vi "Lockstep Move.vi"(6 "Movement Type (0: relative)":u16(ring) items=["relative", "absolute"], 7 "Move Distance (0)":i32, 8 "error in (no error)":errorcluster, 9 "Device Number":string, 10 "Lockstep Group (1)":i32=1, 11 "VISA resource name":refnum<visa-resource-name>) -> (0 "error out":errorcluster, 3 "VISA resource name out":refnum<visa-resource-name>)   [LabVIEW 2018, in "Zaber A Series.lvlib"]
doc: "Moves a lockstep group, which is a collection of axes that move in unison. You can specifiy the type of movement (absolute or relative) and the distance the device's native position units. See your device manual for the unit conversion, or use the Convert Position Units to Device Units VI to convert from standard length units.\n\nNo responses are returned with this VI, but if you would like to wait until the movement is completed to continue, you can combine this VI with the Poll Until Idle VI. \n\nThis VI requires that the Initialize VI has been called with the same serial port and that the lockstep group has been created with the Lockstep Enable VI. \n\nNote: See the Device Lookup control for the microstep size of your model, or check on the product specifications page for the product on www.zaber.com."
uses:
  Zaber A Series.lvlib
  Private/Basic Commands.ctl
  Private/All Commands.ctl
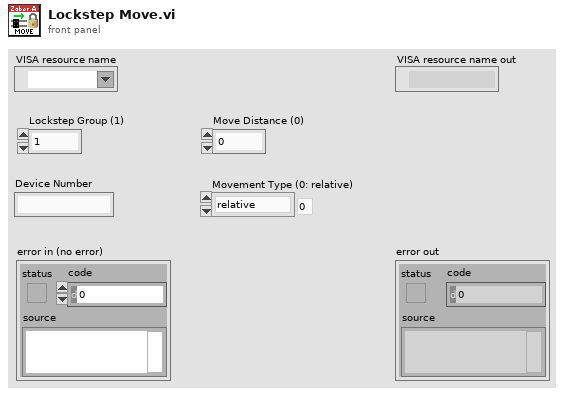
[diagram p1: front panel]
types:
  T1 = typedef "Zaber A Series.lvlib/All Commands.ctl" = string
  T2 = typedef "Zaber A Series.lvlib/Basic Commands.ctl" = string
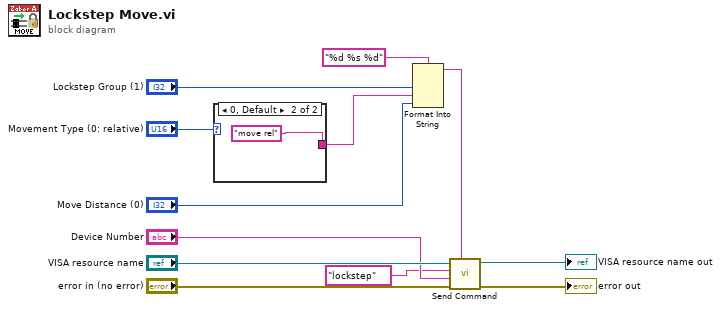
[diagram p0: block diagram]
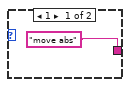
[diagram p2: hidden frame]
diagram:
  n1 = case shown="0, Default" "Movement Type (0: relative)" {
    tunnel: [T2 "move abs" ("Basic Command List") T2 "move rel" ("Basic Command List")] -> w6
    frame 1 {
    }
    frame 0, Default {
    }
  }
  n2 = Format Into String(format string="%d %s %d", "Lockstep Group (1)", w6, "Move Distance (0)") -> (resulting string=w4:string)  [unwired: 2 in, 1 out]
  n3 = call "Send Command.vi"("Data"=w4, "error in (no error)"="error in (no error)", "Device and Axis"="Device Number", "Command"=T1 "lockstep" ("Complete Command List"), "VISA resource name"="VISA resource name") -> ("error out"=→"error out":errorcluster, "VISA resource name out"=→"VISA resource name out":refnum<visa-resource-name>)  [unwired: 1 in, 4 out]
